vi "reql_item_get.vi"(6 "ms timeout (0:default)":i32, 7 "db name":string, 8 "error in (no error)":errorcluster, 9 "id":string, 10 "table name":string, 11 "rethinkdb in":refnum<class "RethinkDB.lvclass">) -> (0 "error out":errorcluster, 2 "value":variant, 3 "rethinkdb out":refnum<class "RethinkDB.lvclass">, 4 "response":variant)   [LabVIEW 2017, in "rethinkdb.lvlib"]
uses:
  rethinkdb.lvlib
  RethinkDB.lvclass
  ql2_query.ctl
  ql2_term.ctl
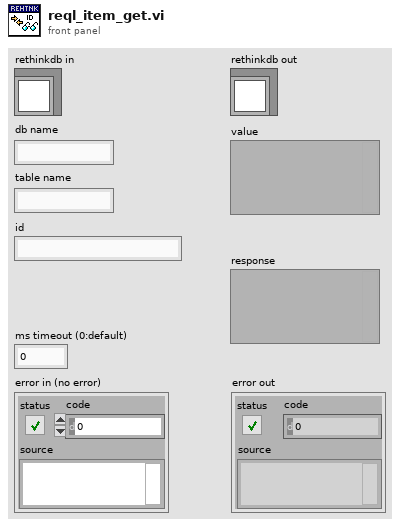
[diagram p1: front panel]
types:
  T1 = typedef "rethinkdb.lvlib/ql2_term.ctl" = enum8{"ADD", "AND", "APPEND", "APRIL", "ARGS", "ASC", "AUGUST", "AVG", "BETWEEN", "BETWEEN_DEPRECATED", "BINARY", "BIT_AND", "BIT_NOT", "BIT_OR", "BIT_SAL", "BIT_SAR", "BIT_XOR", "BRACKET", "BRANCH", "CEIL", "CHANGES", "CHANGE_AT", "CIRCLE", "COERCE_TO", "CONCAT_MAP", "CONFIG", "CONTAINS", "COUNT", "DATE", "DATUM", "DAY", "DAY_OF_WEEK", "DAY_OF_YEAR", "DB", "DB_CREATE", "DB_DROP", "DB_LIST", "DECEMBER", "DEFAULT", "DELETE", "DELETE_AT", "DESC", "DIFFERENCE", "DISTANCE", "DISTINCT", "DIV", "DOWNCASE", "DURING", "EPOCH_TIME", "EQ", "EQ_JOIN", "ERROR", "FEBRUARY", "FILL", "FILTER", "FLOOR", "FOLD", "FOR_EACH", "FRIDAY", "FUNC", "FUNCALL", "GE", "GEOJSON", "GET", "GET_ALL", "GET_FIELD", "GET_INTERSECTING", "GET_NEAREST", "GET_WRITE_HOOK", "GRANT", "GROUP", "GT", "HAS_FIELDS", "HOURS", "HTTP", "IMPLICIT_VAR", "INCLUDES", "INDEX_CREATE", "INDEX_DROP", "INDEX_LIST", "INDEX_RENAME", "INDEX_STATUS", "INDEX_WAIT", "INFO", "INNER_JOIN", "INSERT", "INSERT_AT", "INTERSECTS", "IN_TIMEZONE", "ISO8601", "IS_EMPTY", "JANUARY", "JAVASCRIPT", "JSON", "JULY", "JUNE", "KEYS", "LE", "LIMIT", "LINE", "LITERAL", "LT", "MAKE_ARRAY", "MAKE_OBJ", "MAP", "MARCH", "MATCH", "MAX", "MAXVAL", "MAY", "MERGE", "MIN", "MINUTES", "MINVAL", "MOD", "MONDAY", "MONTH", "MUL", "NE", "NOT", "NOVEMBER", "NOW", "NTH", "OBJECT", "OCTOBER", "OFFSETS_OF", "OR", "ORDER_BY", "OUTER_JOIN", "PLUCK", "POINT", "POLYGON", "POLYGON_SUB", "PREPEND", "RANDOM", "RANGE", "REBALANCE", "RECONFIGURE", "REDUCE", "REPLACE", "ROUND", "SAMPLE", "SATURDAY", "SECONDS", "SEPTEMBER", "SET_DIFFERENCE", "SET_INSERT", "SET_INTERSECTION", "SET_UNION", "SET_WRITE_HOOK", "SKIP", "SLICE", "SPLICE_AT", "SPLIT", "STATUS", "SUB", "SUM", "SUNDAY", "SYNC", "TABLE", "TABLE_CREATE", "TABLE_DROP", "TABLE_LIST", "THURSDAY", "TIME", "TIMEZONE", "TIME_OF_DAY", "TO_EPOCH_TIME", "TO_GEOJSON", "TO_ISO8601", "TO_JSON_STRING", "TUESDAY", "TYPE_OF", "UNGROUP", "UNION", "UPCASE", "UPDATE", "UUID", "VALUES", "VAR", "WAIT", "WEDNESDAY", "WITHOUT", "WITH_FIELDS", "YEAR", "ZIP", "invalid"}
  T2 = typedef "rethinkdb.lvlib/ql2_query.ctl" = enum8{"START", "CONTINUE", "STOP", "NOREPLY_WAIT", "SERVER_INFO", "invalid"}
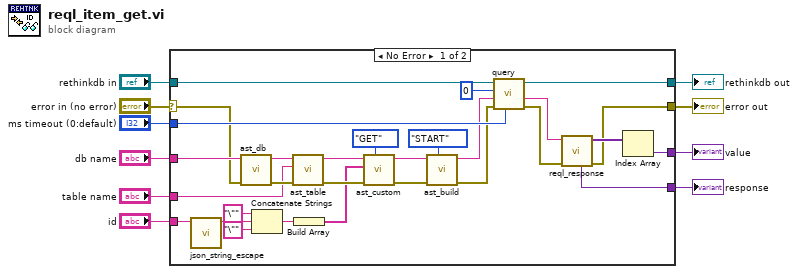
[diagram p0: block diagram]
diagram:
  n1 = case shown="No Error" "error in (no error)" {
    selector: "error in (no error)" -> [w28 w41]
    tunnel: "rethinkdb in" -> [w33 w40]
    tunnel: [w39 w40] -> w8
    tunnel: "ms timeout (0:default)" -> [w38 _]
    tunnel: [w17 w41] -> w6
    tunnel: "db name" -> [w32 _]
    tunnel: "table name" -> [w29 _]
    tunnel: [w24 _] -> w3
    tunnel: "id" -> [w12 _]
    tunnel: [w16 _] -> w1
    frame No Error {
      n2 = call "json_string_escape.vi"("string"=w12) -> ("escaped string"=w15:string)  [unwired: 10 in]
      n3 = call "ast_db.vi"("error in (no error)"=w28, "db name"=w32) -> ("error out"=w30:errorcluster, "r.db"=w31:string)  [unwired: 8 in]
      n4 = Concatenate Strings("\"" ("string"), w15, "\"" ("string")) -> (w11:string)
      n5 = call "ast_table.vi"("error in (no error)"=w30, "table name"=w29, "r.db"=w31) -> ("error out"=w23:errorcluster, "r.db.table"=w21:string)  [unwired: 7 in]
      n6 = Build Array(w11) -> (w19:string[])
      n7 = call "ast_custom.vi"("term_type"=ql2_term."GET", "error in (no error)"=w23, "args"=w19, "arg0"=w21) -> ("error out"=w22:errorcluster, "r"=w20:string)  [unwired: 6 in]
      n8 = call "ast_build.vi"("query_type"=ql2_query."START", "error in (no error)"=w22, "term"=w20) -> ("error out"=w27:errorcluster, "query"=w26:string)  [unwired: 7 in]
      n9 = call "query.vi"("ms timeout (0:default)"=w38, "error in (no error)"=w27, "query"=w26, "token in (random)"=u64 0, "rethinkdb in"=w33) -> ("error out"=w36:errorcluster, "response"=w35:string, "rethinkdb out"=w39:refnum<class "RethinkDB.lvclass">)  [unwired: 3 in, 1 out]
      n10 = call "reql_response.vi"("error in (no error)"=w36, "response"=w35) -> ("error out"=w17:errorcluster, "values"=w34:variant[], "response"=w24:variant)  [unwired: 7 in]
      n11 = Index Array(array=w34) -> (element=w16:variant)  [unwired: 1 in]
    }
    frame Error {
    }
  }
  "error out" <- w6
  "rethinkdb out" <- w8
  "response" <- w3
  "value" <- w1
